vi "Test Stop Nested Actors.vi"(8 "error in":errorcluster, 11 "Test Case In":refnum<class "Nested Actor.lvclass">) -> (0 "error out":errorcluster, 3 "Test Case Out":refnum<class "Nested Actor.lvclass">)   [LabVIEW 2020, in "Nested Actor.lvclass"]
uses:
  Nested Actor.lvclass
  C:/Program Files/National Instruments/LabVIEW 2024/vi.lib/Astemes/LUnit/Test Case.lvclass
  Actor with Nesteds/Actor with Nesteds/Actor with Nesteds.lvclass
  C:/Users/J63553/Projects/_LabVIEW Community/actor-framework/Core/ActorFramework/Actor/Actor.lvclass
  Core/ActorFramework/Message Queue/Message Queue.lvclass/Message Queue.ctl
  Core/ActorFramework/Message Enqueuer/Message Enqueuer.lvclass/Message Enqueuer.ctl
  Core/ActorFramework/Message Dequeuer/Message Dequeuer.lvclass/Message Dequeuer.ctl
  <vilib>/Astemes/LUnit/Test Case.lvclass/Test Case.ctl
  f6bf6e7a-8cea-4d98-973d-9df0f0475c28.vi
  Core/ActorFramework/Message Enqueuer/Enqueue.vi
  <vilib>/Astemes/LUnit/Append Pass Result.vi
  <vilib>/Astemes/LUnit/Append Fail Result.vi
  f6bf6e7a-8cea-4d98-973d-9df0f0475c28.vi/9c5d11cd-9439-4240-a1ee-d9baace9c924.vi
  <vilib>/Astemes/LUnit/Run In UI.vi
  <vilib>/Utility/error.llb/Clear Errors.vi
  Actor with Nesteds/Stop Nested Actors Msg/Stop Nested Actors Msg.lvclass
  C:/Users/J63553/Projects/_LabVIEW Community/actor-framework/Core/ActorFramework/Message/Message.lvclass
  Core/ActorFramework/Stop Msg/Stop Msg.lvclass
  Core/ActorFramework/Message Priority Queue/Priority Enqueue.vi
  Core/ActorFramework/Message Priority Queue/Priority Dequeue.vi
  Core/ActorFramework/Actor/Actor.lvclass
  Core/ActorFramework/Message Queue/Message Queue.lvclass
  Core/ActorFramework/Message Dequeuer/Message Dequeuer.lvclass
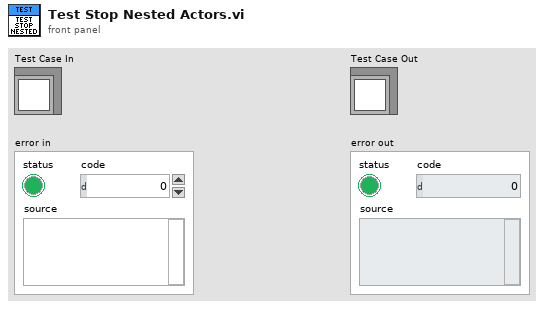
[diagram p1: front panel]
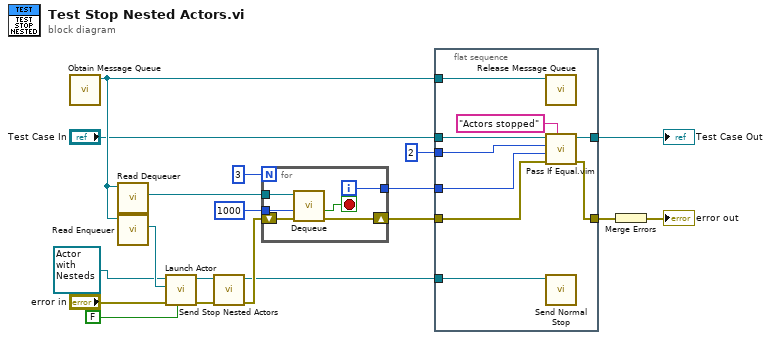
[diagram p0: block diagram]
diagram:
  n1 = call "Obtain Message Queue.vi"() -> ("Message Queue"=w8:refnum<class "Message Queue.lvclass">)  [unwired: 10 in, 1 out]
  n2 = call "Read Dequeuer.vi"("Message Queue"=w8) -> ("Message Dequeuer"=w10:refnum<class "Message Dequeuer.lvclass">)  [unwired: 10 in]
  n3 = call "Read Enqueuer.vi"("Message Queue"=w8) -> ("Message Enqueuer"=w13:refnum<class "Message Enqueuer.lvclass">)  [unwired: 10 in]
  n4 = call "Launch Actor.vi"("Open Actor Core front panel? (F)"=FALSE, "error in (no error)"="error in", "Actor-to-Caller Enqueuer"=w13, "Actor"=refnum<class "Actor with Nesteds.lvclass"> refnum ("Actor with Nesteds.lvlib:Actor with Nesteds.lvclass")) -> ("error out"=w18:errorcluster, "Caller-To-Actor Enqueuer"=w12:refnum<class "Message Enqueuer.lvclass">)  [unwired: 6 in]
  n5 = call "Send Stop Nested Actors.vi"("error in (no error)"=w18, "Message Enqueuer"=w12) -> ("error out"=w17:errorcluster, "Message Enqueuer out"=w3:refnum<class "Message Enqueuer.lvclass">)  [unwired: 8 in]
  n6 = for {
    N: 3 -> [_]
    tunnel: 1000 ("milliseconds to wait") -> [w23]
    tunnel: w10 -> [w22]
    shift-right: [w24] -> w16
    shift-left: w17 -> [w25]
    tunnel: [w20] -> w5
    i -> [w20]
    stop <- w21 stop-if-true
    n7 = call "Dequeue.vi"("error in (no error)"=w25, "timeout in ms (-1)"=w23, "Message Dequeuer in"=w22) -> ("error out"=w24:errorcluster, "timed out?"=w21:bool)  [unwired: 4 in, 3 out]
  }
  n8 = flat-sequence {
    tunnel: [w34] -> w19
    tunnel: w16 -> [w33]
    tunnel: w8 -> [w32]
    tunnel: w5 -> [w28]
    tunnel: 2 -> [w29]
    tunnel: w3 -> [w31]
    tunnel: "Test Case In" -> [w27]
    tunnel: [w26] -> w1
    frame #0 {
      n9 = call "Release Message Queue.vi"("Message Queue"=w32) -> ()  [unwired: 9 in, 2 out]
      n10 = call "Pass If Equal.vim"("Description"="Actors stopped" ("Label (VI Title)"), "error in (no error)"=w33, "Actual"=w28, "Expected"=w29, "LUnit Test Case In"=w27) -> ("error out"=w34:errorcluster, "LUnit Test Case Out"=w26:refnum<class "Nested Actor.lvclass">)  [unwired: 5 in]
      n11 = call "Send Normal Stop.vi"("Message Enqueuer"=w31) -> ()  [unwired: 10 in, 1 out]
    }
  }
  n12 = Merge Errors(w19) -> (→"error out":errorcluster)
  "Test Case Out" <- w1
